vi "From WAMP message code value.vi"(8 "error IO":errorcluster, 9 "WAMP Numeric value":u8) -> (2 "error out":errorcluster, 3 "Message Type":T1)   [LabVIEW 2020, in "wamplv.lvlib"]
uses:
  wamplv.lvlib
  TypeDefs/WAMP Message Codes.ctl
  <vilib>/Utility/error.llb/Error Cluster From Error Code.vi
  <vilib>/ErrorRing/Error Ring.xnode
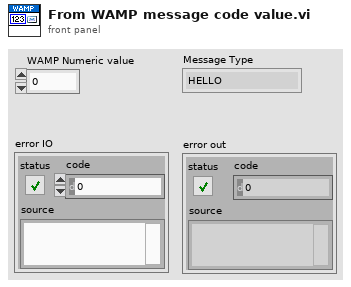
[diagram p1: front panel]
types:
  T1 = typedef "wamplv.lvlib/WAMP Message Codes.ctl" = enum8{"HELLO", "WELCOME", "ABORT", "GOODBYE", "ERROR", "PUBLISH", "PUBLISHED", "SUBSCRIBE", "SUBSCRIBED", "UNSUBSCRIBE", "UNSUBSCRIBED", "EVENT", "CALL", "RESULT", "REGISTER", "REGISTERED", "UNREGISTER", "UNREGISTERED", "INVOCATION", "YIELD"}
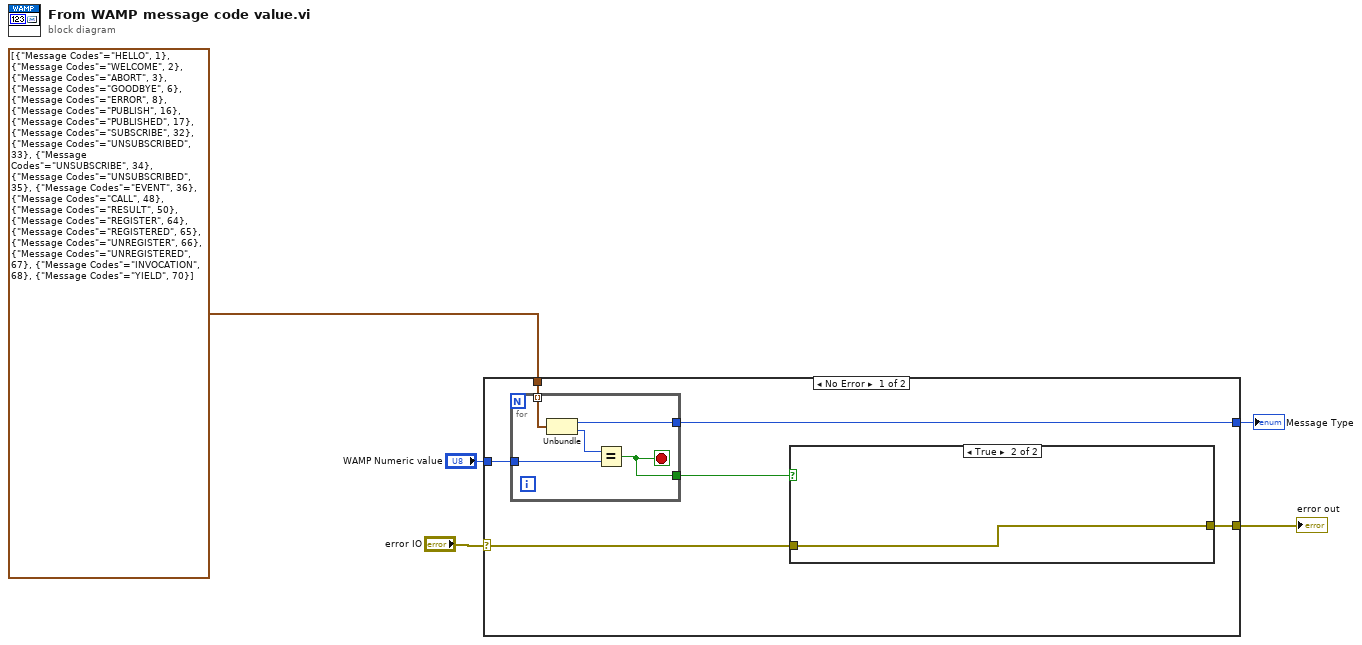
[diagram p0: block diagram]
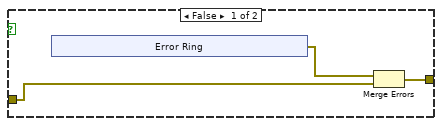
[diagram p2: hidden frame]
diagram:
  n1 = case shown="No Error" "error IO" {
    selector: "error IO" -> [w7 w25]
    tunnel: cluster{"Message Codes":T1, u8}[] [{"Message Codes"=enum."HELLO", 1}, {"Message Codes"=enum."WELCOME", 2}, {"Message Codes"=enum."ABORT", 3}, {"Message Codes"=enum."GOODBYE", 6}, {"Message Codes"=enum."ERROR", 8}, {"Message Codes"=enum."PUBLISH", 16}, {"Message Codes"=enum."PUBLISHED", 17}, {"Message Codes"=enum."SUBSCRIBE", 32}, {"Message Codes"=enum."UNSUBSCRIBED", 33}, {"Message Codes"=enum."UNSUBSCRIBE", 34}, {"Message Codes"=enum."UNSUBSCRIBED", 35}, {"Message Codes"=enum."EVENT", 36}, {"Message Codes"=enum."CALL", 48}, {"Message Codes"=enum."RESULT", 50}, {"Message Codes"=enum."REGISTER", 64}, {"Message Codes"=enum."REGISTERED", 65}, {"Message Codes"=enum."UNREGISTER", 66}, {"Message Codes"=enum."UNREGISTERED", 67}, {"Message Codes"=enum."INVOCATION", 68}, {"Message Codes"=enum."YIELD", 70}] ("output cluster") -> [w11 _]
    tunnel: "WAMP Numeric value" -> [w10 _]
    tunnel: [w8 _] -> w3
    tunnel: [w6 w25] -> w1
    frame No Error {
      n2 = for {
        tunnel: w11 -> [w24] mode=indexing
        tunnel: w10 -> [w20]
        tunnel: [w23] -> w8
        tunnel: [w22] -> w9
        stop <- w22 stop-if-true
        n3 = Unbundle(w24) -> ("Message Codes"=w23:T1, w21:u8)
        n4 = Equal?(x=w21, y=w20) -> (x = y?=w22:bool)
      }
      n5 = case shown="True" w9 {
        tunnel: w7 -> [w13 w19]
        tunnel: [w12 w19] -> w6
        frame False {
          n6 = xnode "Error Ring"() -> ("error out"=w14:errorcluster)
          n7 = Merge Errors(w14, w13) -> (w12:errorcluster)
        }
        frame True {
        }
      }
    }
    frame Error {
    }
  }
  "Message Type" <- w3
  "error out" <- w1
